vi "模拟输入_电阻_连续.vi"() -> ()   [LabVIEW 2013]
doc: "This example demonstrates how to acquire a continuous data."
uses:
  <userlib>/ArtDAQ/_SubVI/ArtDAQ_CreateAIResistanceChan.vi
  <userlib>/ArtDAQ/_SubVI/ArtDAQ_CfgSampClkTiming.vi
  <userlib>/ArtDAQ/_SubVI/ArtDAQ_Read Analog DBL NChan NSamp.vi
panel:
  in  "电流激励值":dbl=0.004 format="%0.3f"
  in  "电流激励源":i32(ring)=10167 items=["内部"=10200, "外部"=10167, "无"=10230]
  in  "电阻配置":i32(ring)=2 items=["2-线"=2, "3-线"=3, "4-线"=4]
  in  "最大值":dbl=1000.0 format="%.2f"
  in  "最小值":dbl=100.0 format="%.2f"
  in  "停止":bool
  out "Waveform":dbl[][](graph)
  in  "采样频率":dbl=10000.0 format="%#_13g"
  in  "每通道采样点数":i32=1000
  in  "物理通道":string(combo)="Dev1/ai0"
  out "错误":errorcluster
  # "通道属性"
  # "定时"
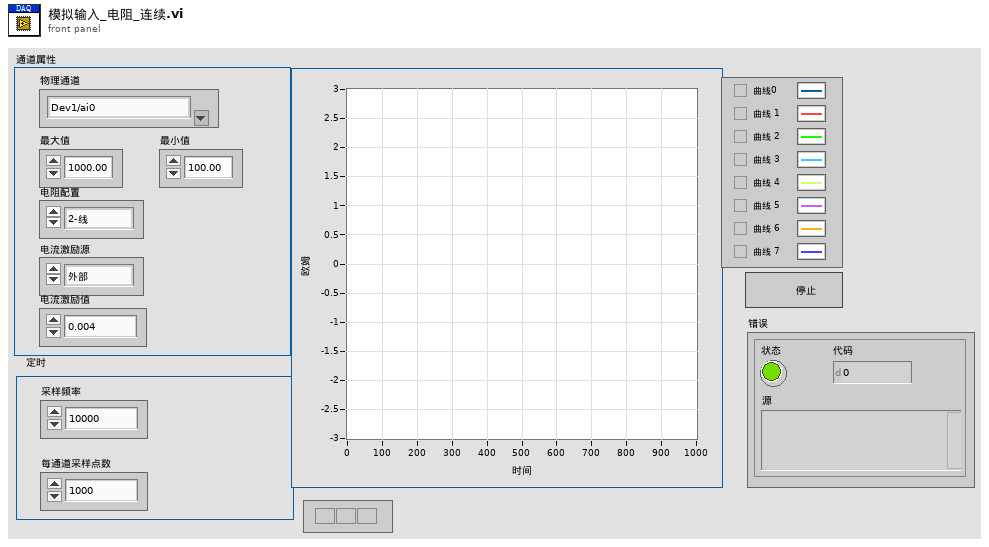
[diagram p1: front panel]
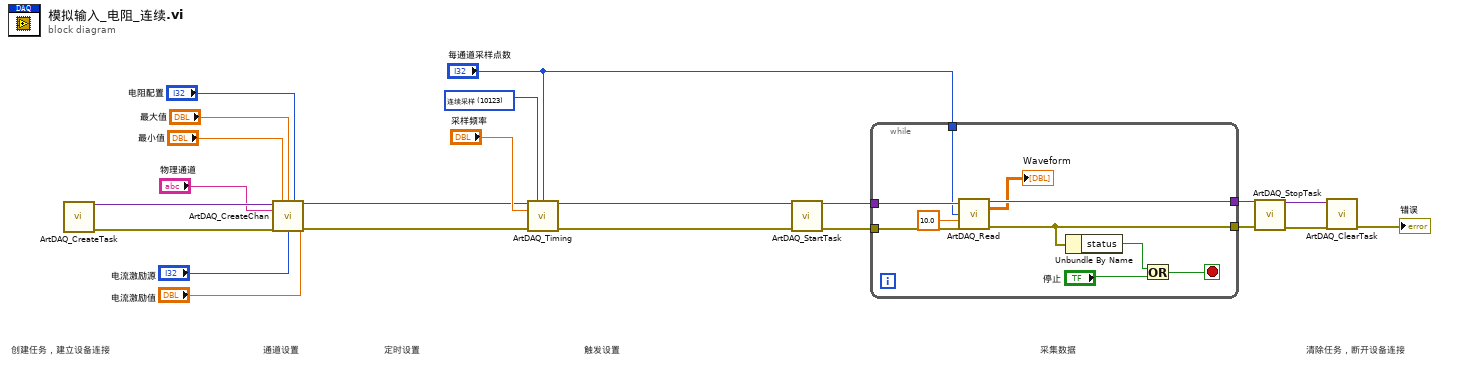
[diagram p0: block diagram]
diagram:
  w8 = 10123 items=["有限点采样"=10178, "连续采样"=10123] ("SampleMode")
  # "清除任务，断开设备连接"
  # "采集数据"
  # "触发设置"
  # "定时设置"
  # "通道设置"
  # "创建任务，建立设备连接"
  n1 = call <userlib>:"ArtDAQ_CreateTask.vi"() -> ("任务句柄"=w15:variant, "错误输出"=w22:errorcluster)  [unwired: 14 in]
  n2 = call-poly <userlib>:"ArtDAQ_CreateChan.vi"("任务句柄"=w15, "最小值"="最小值", "最大值"="最大值", "电阻配置"="电阻配置", "物理通道"="物理通道", "电流激励值"="电流激励值", "错误输入"=w22, "电流激励源"="电流激励源") -> ("任务句柄"=w9:variant, "错误输出"=w21:errorcluster)  [unwired: 6 in]
  n3 = call-poly <userlib>:"ArtDAQ_Timing.vi"("任务句柄"=w9, "采样模式"=w8, "每通道采样数"="每通道采样点数", "采样率"="采样频率", "错误输入"=w21) -> ("任务句柄"=w7:variant, "错误输出"=w6:errorcluster)  [unwired: 9 in]
  n4 = call <userlib>:"ArtDAQ_StartTask.vi"("任务句柄"=w7, "错误输入"=w6) -> ("任务句柄"=w18:variant, "错误输出"=w17:errorcluster)  [unwired: 12 in]
  n5 = while {
    tunnel: w18 -> [w32]
    tunnel: w17 -> [w31]
    tunnel: "每通道采样点数" -> [w30]
    tunnel: [w28] -> w14
    tunnel: [w27] -> w13
    stop <- w25 stop-if-true
    n6 = call-poly <userlib>:"ArtDAQ_Read.vi"("任务句柄"=w32, "每通道采样数"=w30, "超时s"=10.0 ("Timeout"), "错误输入"=w31) -> ("任务句柄"=w28:variant, "数据"=→"Waveform":dbl[][], "错误输出"=w27:errorcluster)  [unwired: 8 in, 1 out]
    n7 = Unbundle By Name(w27) -> ("status"=w26:bool)
    n8 = Or(x=w26, y="停止") -> (x .or. y?=w25:bool)
  }
  n9 = call <userlib>:"ArtDAQ_StopTask.vi"("任务句柄"=w14, "错误输入"=w13) -> ("任务句柄"=w12:variant, "错误输出"=w11:errorcluster)  [unwired: 12 in]
  n10 = call <userlib>:"ArtDAQ_ClearTask.vi"("任务句柄"=w12, "错误输入"=w11) -> ("错误输出"=→"错误":errorcluster)  [unwired: 13 in]
